vi "Create Jerk.vi"(0 "Rise time (ms)":dbl, 7 "Sampling Rate (Hz)":dbl, 9 "Npts":i32, 11 "error in (no error)":errorcluster) -> (4 "Waveform":dbl[](array[numeric]), 15 "error out":errorcluster)   [LabVIEW 2020]
uses:
  <vilib>/Analysis/1siggen.llb/Ramp Pattern by Samples.vi
  <vilib>/Analysis/NI_AALBase.lvlib
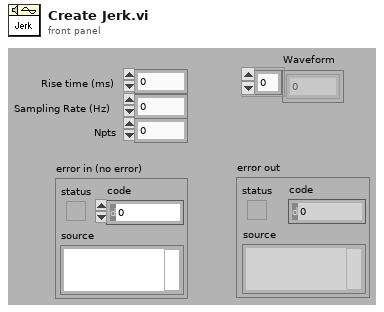
[diagram p1: front panel]
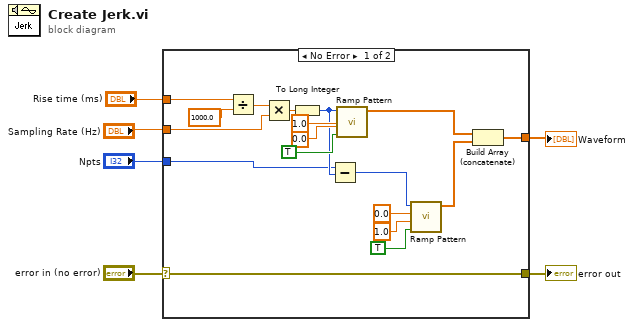
[diagram p0: block diagram]
diagram:
  n1 = case shown="No Error" "error in (no error)" {
    selector: "error in (no error)" -> [w24 w25]
    tunnel: [w24 w25] -> w5
    tunnel: "Sampling Rate (Hz)" -> [w21 _]
    tunnel: "Npts" -> [w8 _]
    tunnel: [w9 _] -> w3
    tunnel: "Rise time (ms)" -> [w7 _]
    frame No Error {
      n2 = Divide(x=w7, y=1000.0) -> (x/y=w22:dbl)
      n3 = Multiply(x=w22, y=w21) -> (x*y=w20:dbl)
      n4 = To Long Integer(number=w20) -> (32bit integer=w13:i32)
      n5 = Subtract(x=w8, y=w13) -> (x-y=w12:i32)
      n6 = call-poly <vilib>:"Ramp Pattern.vi"("exclude end?"=TRUE, "start"=0.0, "end"=1.0, "samples"=w13) -> ("Ramp Pattern"=w11:dbl[])  [unwired: 6 in, 1 out]
      n7 = call-poly <vilib>:"Ramp Pattern.vi"("exclude end?"=TRUE, "start"=1.0, "end"=0.0, "samples"=w12) -> ("Ramp Pattern"=w10:dbl[])  [unwired: 6 in, 1 out]
      n8 = Build Array (concatenate)(w11, w10) -> (w9:dbl[])
    }
    frame Error {
    }
  }
  "error out" <- w5
  "Waveform" <- w3
